vi "Divisor de corrente.vi"() -> ()   [LabVIEW 2014]
uses:
  <vilib>/imath/engines/lvmath2/RunTimeEngine/NodeEndStatement/NIMS_NodeEndStatement_Output.vi
  <instcachedir>/0/NIMS_NodeEndStatement_Output_53EC0D466D134D7ABD903AC30B43404B.lvgen/NIMS_NodeEndStatement_Output_53EC0D466D134D7ABD903AC30B43404B_001.vi
  <vilib>/imath/engines/lvmath2/RunTimeEngine/ErrorHandling/NIMS_Finalize Error.vi
panel:
  in  "R1":dbl
  in  "R2":dbl
  in  "R3":dbl
  in  "stop":bool
  out "IR3":dbl
  out "IR2":dbl
  out "IR1":dbl
  in  "Fonte (A)":dbl
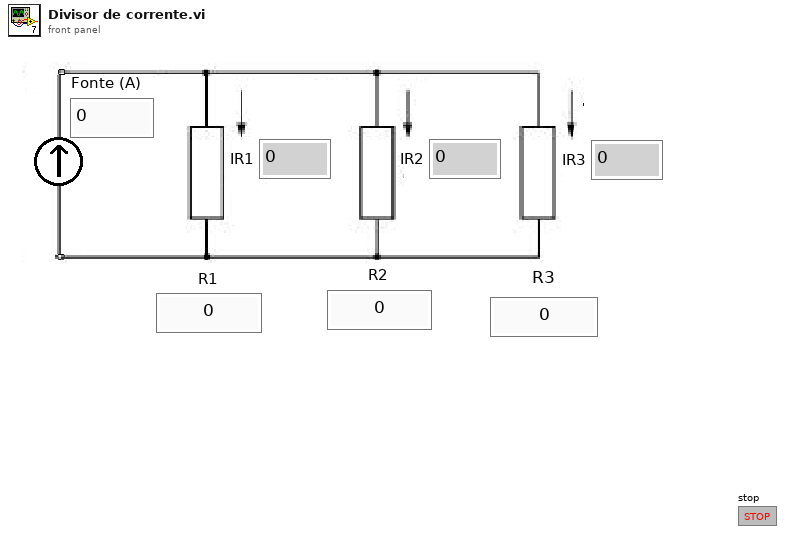
[diagram p1: front panel]
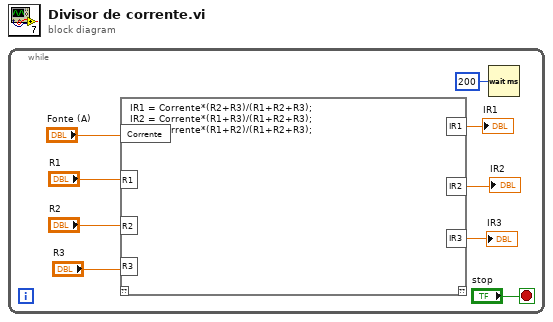
[diagram p0: block diagram]
diagram:
  n1 = while {
    stop <- "stop" stop-if-true
    n2 = mathscript code="IR1 = Corrente*(R2+R3)/(R1+R2+R3);\nIR2 = Corrente*(R1+R3)/(R1+R2+R3);\nIR3 = Corrente*(R1+R2)/(R1+R2+R3);"("Corrente"="Fonte (A)", "R1"="R1", "R2"="R2", "R3"="R3") -> ("IR1"=→"IR1":dbl, "IR2"=→"IR2":dbl, "IR3"=→"IR3":dbl)  [unwired: 1 in, 1 out]
    n3 = Wait (ms)(milliseconds to wait=u32 200) -> ()  [unwired: 1 out]
  }
